vi "Experiment2_Init.vi"(0 "object in":refnum<class "Experiment2.lvclass">, 1 "DOClockSettings":T3, 2 "Sequence Settings":T4, 3 "WFGConfig":T5={"Running"=FALSE, "Ch1"={"idxChannel"=0, "Settings out of range"=FALSE, "Carrier"={"Frequency (Hz)"=1000.0, "Amplitude (V)"=1.0, "Offset(V)"=0.0, "Symmetry(%) "=50.0, "Phase(Deg)"=0.0, "Function"=1, "Enable"=TRUE}, "Trigger"={"secRun(0=Cont)"=0.0, "secWait"=0.0, "cRepeat(0=inf)"=0, "Repeat Trigger"=FALSE, "TrigrSrc"=enum."trigrsrcNone"}, "FM Mod"={"Frequency (Hz)"=1000.0, "Amplitude (%)"=1.0, "Offset(V)"=0.0, "Symmetry(%) "=50.0, "Phase(Deg)"=0.0, "Function 2"=1, "Enable"=FALSE}}, "Ch2"={"idxChannel"=0, "Settings out of range"=FALSE, "Carrier"={"Frequency (Hz)"=1000.0, "Amplitude (V)"=1.0, "Offset(V)"=0.0, "Symmetry(%) "=50.0, "Phase(Deg)"=0.0, "Function"=1, "Enable"=TRUE}, "Trigger"={"secRun(0=Cont)"=0.0, "secWait"=0.0, "cRepeat(0=inf)"=0, "Repeat Trigger"=FALSE, "TrigrSrc"=enum."trigrsrcNone"}, "FM Mod"={"Frequency (Hz)"=1000.0, "Amplitude (%)"=1.0, "Offset(V)"=0.0, "Symmetry(%) "=50.0, "Phase(Deg)"=0.0, "Function 2"=1, "Enable"=FALSE}}, "SyncronizeState"=enum."Independent"} {"Ch2"."FM Mod"."Function 2" items=["DC"=0, "Sine"=1, "Square"=2, "Triangle"=3, "RampUp"=4, "RampDown"=5, "Noise"=6, "Pulse"=7, "Custom"=30]; "Ch2"."Carrier"."Function" items=["DC"=0, "Sine"=1, "Square"=2, "Triangle"=3, "RampUp"=4, "RampDown"=5, "Noise"=6, "Pulse"=7, "Custom"=30]; "Ch1"."FM Mod"."Function 2" items=["DC"=0, "Sine"=1, "Square"=2, "Triangle"=3, "RampUp"=4, "RampDown"=5, "Noise"=6, "Pulse"=7, "Custom"=30]; "Ch1"."Carrier"."Function" items=["DC"=0, "Sine"=1, "Square"=2, "Triangle"=3, "RampUp"=4, "RampDown"=5, "Noise"=6, "Pulse"=7, "Custom"=30]}, 4 "Repeat ID":dbl, 5 "error in (no error)":errorcluster, 9 "ExperimentFolder":path) -> (14 "object out":refnum<class "Experiment2.lvclass">, 19 "error out":errorcluster)   [LabVIEW 2023, in "Experiment2.lvclass"]
uses:
  Experiment2.lvclass
  AD2_WFG_SDK_class/WFG.ctl
  AD2_WFG_SDK_class/WFGCh.ctl
  AD2_WFG_SDK_class/AD2TriggerSources.ctl
  Experiment2.lvclass/Experiment2.ctl
  AD2_SDK_class/AD2_SDK.lvclass
  AD2_WFG_SDK_class/AD2_WFG_SDK.lvclass
  AD2_DO_SDK_class/DOTrigger.ctl
  AD2_DO_SDK_class/AD2_DO_SDK.lvclass
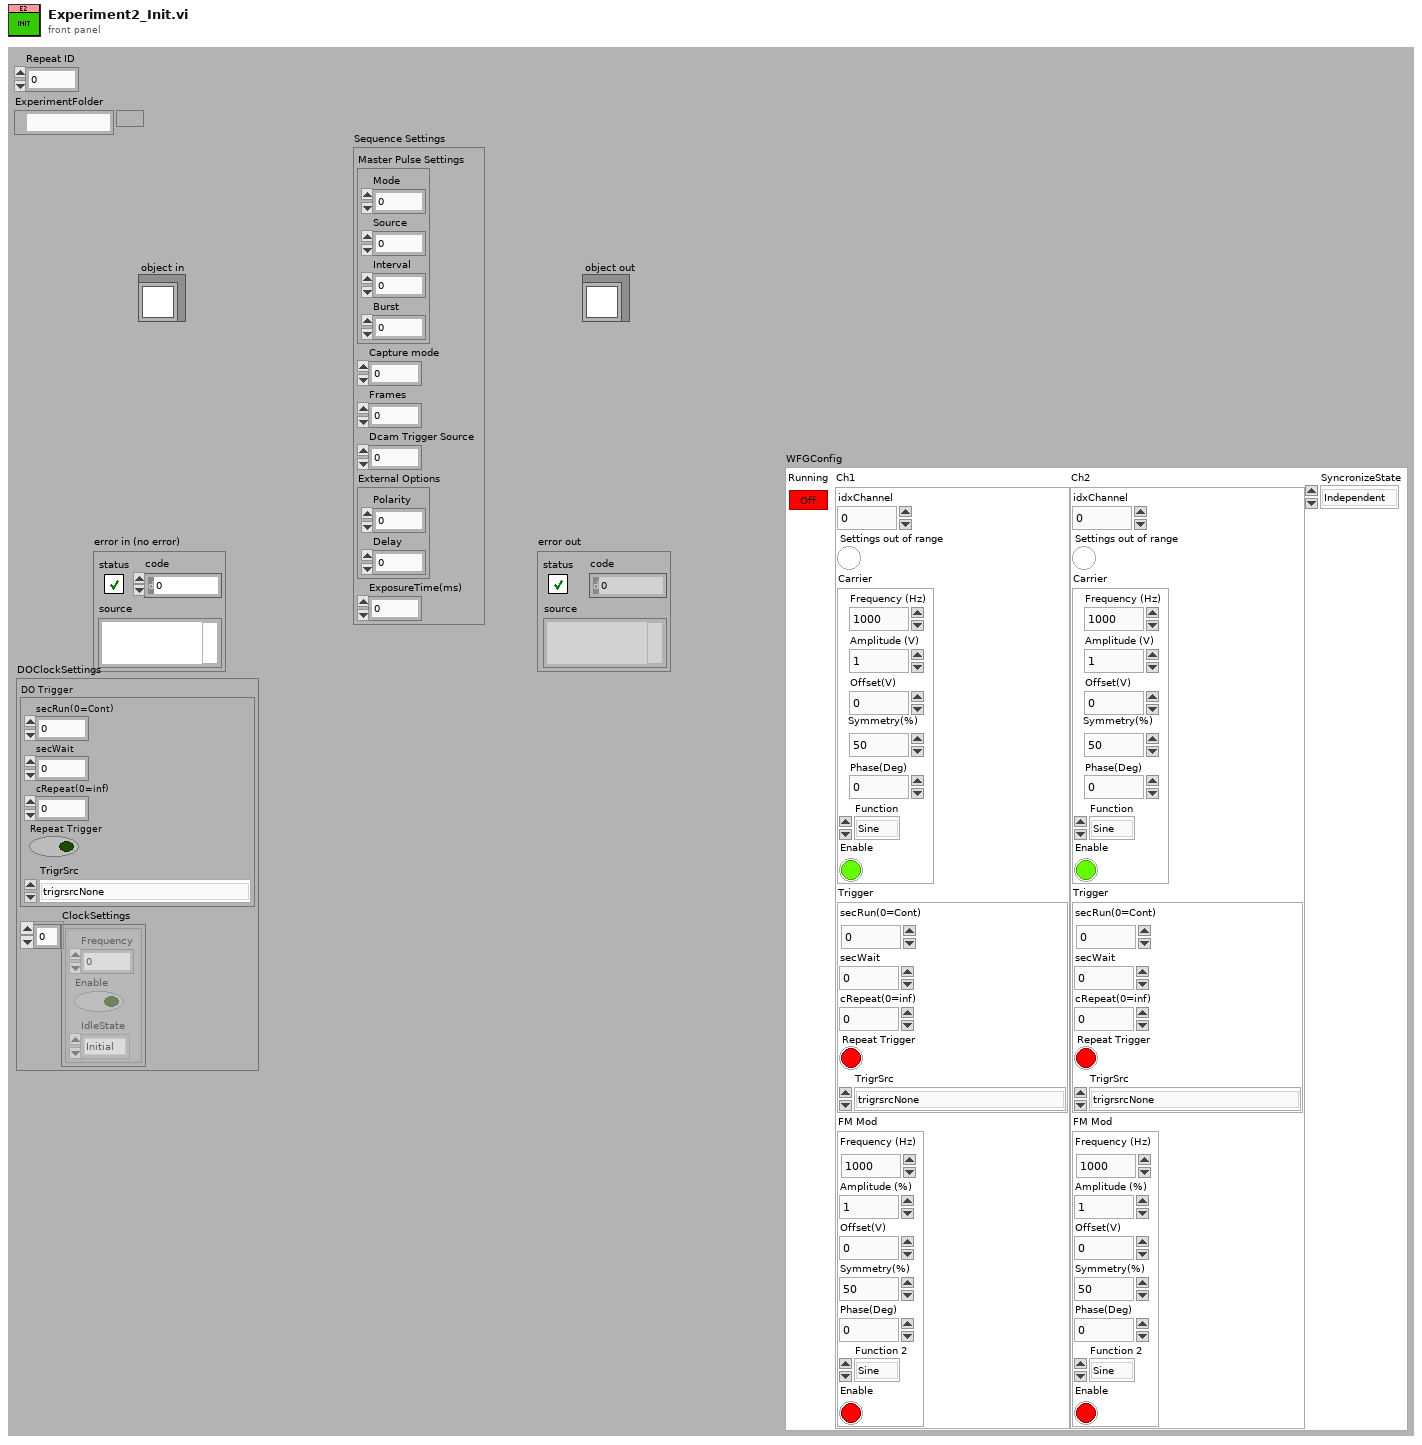
[diagram p1: front panel]
types:
  T1 = typedef "AD2_DO_SDK.lvclass/DOTrigger.ctl" = cluster{"secRun(0=Cont)":dbl, "secWait":dbl, "cRepeat(0=inf)":i32, "Repeat Trigger":bool, "TrigrSrc":T2}
  T2 = typedef "AD2_SDK.lvclass/AD2TriggerSources.ctl" = enum8{"trigrsrcNone", "trigsrcPC", "trigsrcDetectorAnalogIn", "trigsrcDetectorDigitalIn", "trigsrcAnalogIn", "trigsrcDigitalIn", "trigsrcDigitalOut", "trigsrcAnalogOut1", "trigsrcAnalogOut2", "trigsrcAnalogOut3", "trigsrcAnalogOut4", "trigsrcExternal1", "trigsrcExternal2", "trigsrcExternal3", "trigsrcExternal4", ""}
  T3 = cluster{"DO Trigger":T1, "ClockSettings":cluster{"Frequency":dbl, "Enable":bool, "IdleState":enum16{"Initial", "Low", "High", "Z"}}[]}
  T4 = cluster{"Master Pulse Settings":cluster{"Mode":u32, "Source":u32, "Interval":dbl, "Burst":u32}, "Capture mode":i32, "Frames":i32, "Dcam Trigger Source":i32, "External Options":cluster{"Polarity":i32, "Delay":dbl}, "ExposureTime(ms)":dbl}
  T5 = typedef "AD2_WFG_SDK.lvclass/WFG.ctl" = cluster{"Running":bool, "Ch1":T6, "Ch2":T6, "SyncronizeState":enum16{"Independent", "Ch1Master", "Ch2Master"}}
  T6 = typedef "AD2_WFG_SDK.lvclass/WFGCh.ctl" = cluster{"idxChannel":i32, "Settings out of range":bool, "Carrier":cluster{"Frequency (Hz)":dbl, "Amplitude (V)":dbl, "Offset(V)":dbl, "Symmetry(%) ":dbl, "Phase(Deg)":dbl, "Function":u16, "Enable":bool}, "Trigger":cluster{"secRun(0=Cont)":dbl, "secWait":dbl, "cRepeat(0=inf)":i32, "Repeat Trigger":bool, "TrigrSrc":T2}, "FM Mod":cluster{"Frequency (Hz)":dbl, "Amplitude (%)":dbl, "Offset(V)":dbl, "Symmetry(%) ":dbl, "Phase(Deg)":dbl, "Function 2":u16, "Enable":bool}}
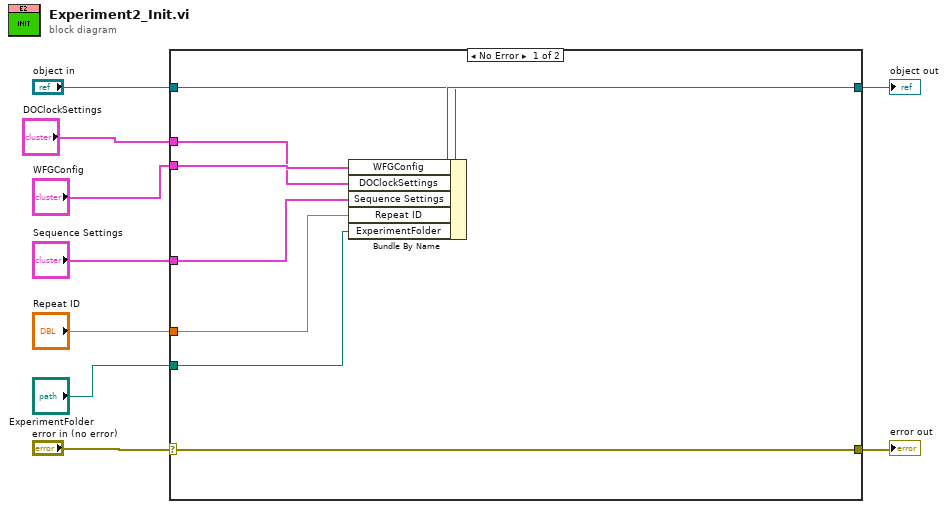
[diagram p0: block diagram]
diagram:
  n1 = case shown="No Error" "error in (no error)" {
    selector: "error in (no error)" -> [w17 w18]
    tunnel: "object in" -> [w15 w19]
    tunnel: [w16 w19] -> w8
    tunnel: [w17 w18] -> w6
    tunnel: "WFGConfig" -> [w14 _]
    tunnel: "Sequence Settings" -> [w13 _]
    tunnel: "Repeat ID" -> [w12 _]
    tunnel: "ExperimentFolder" -> [w11 _]
    tunnel: "DOClockSettings" -> [w10 _]
    frame No Error {
      n2 = Bundle By Name(cluster=w15, "WFGConfig"=w14, "DOClockSettings"=w10, "Sequence Settings"=w13, "Repeat ID"=w12, "ExperimentFolder"=w11) -> (w16:refnum<class "Experiment2.lvclass">)
    }
    frame Error {
    }
  }
  "object out" <- w8
  "error out" <- w6
